vi "Execute.vi"(4 "Position":i32, 6 "Assembly Type":string, 8 "Error In":errorcluster, 9 "Workspace":T1, 10 "Control In":T2={"I-O.lvclass"=refnum, "Gantry"=refnum, "Dispenser"="COM1"}, 11 "Dispense in":refnum<class "Dispense.lvclass">) -> (0 "Error Out":errorcluster, 2 "Control Out":T2={"I-O.lvclass"=refnum, "Gantry"=refnum, "Dispenser"="COM1"}, 3 "Dispense out":refnum<class "Dispense.lvclass">)   [LabVIEW 2021, in "Dispense.lvclass"]
uses:
  Dispense.lvclass
  Controller/Controllers.ctl
  Controller/I-O/I-O.lvclass
  C:/Program Files (x86)/Aerotech/A3200/LabVIEW/2010/Bin/Aerotech.A3200.dll
  Program Files (x86)/Aerotech/A3200/LabVIEW/2010/Bin/Aerotech.A3200.dll
  Workspace/Workspace.ctl
  Dispense.lvclass/Dispense.ctl
  Controller/Controller.lvclass
  Workspace/Fixture.lvclass
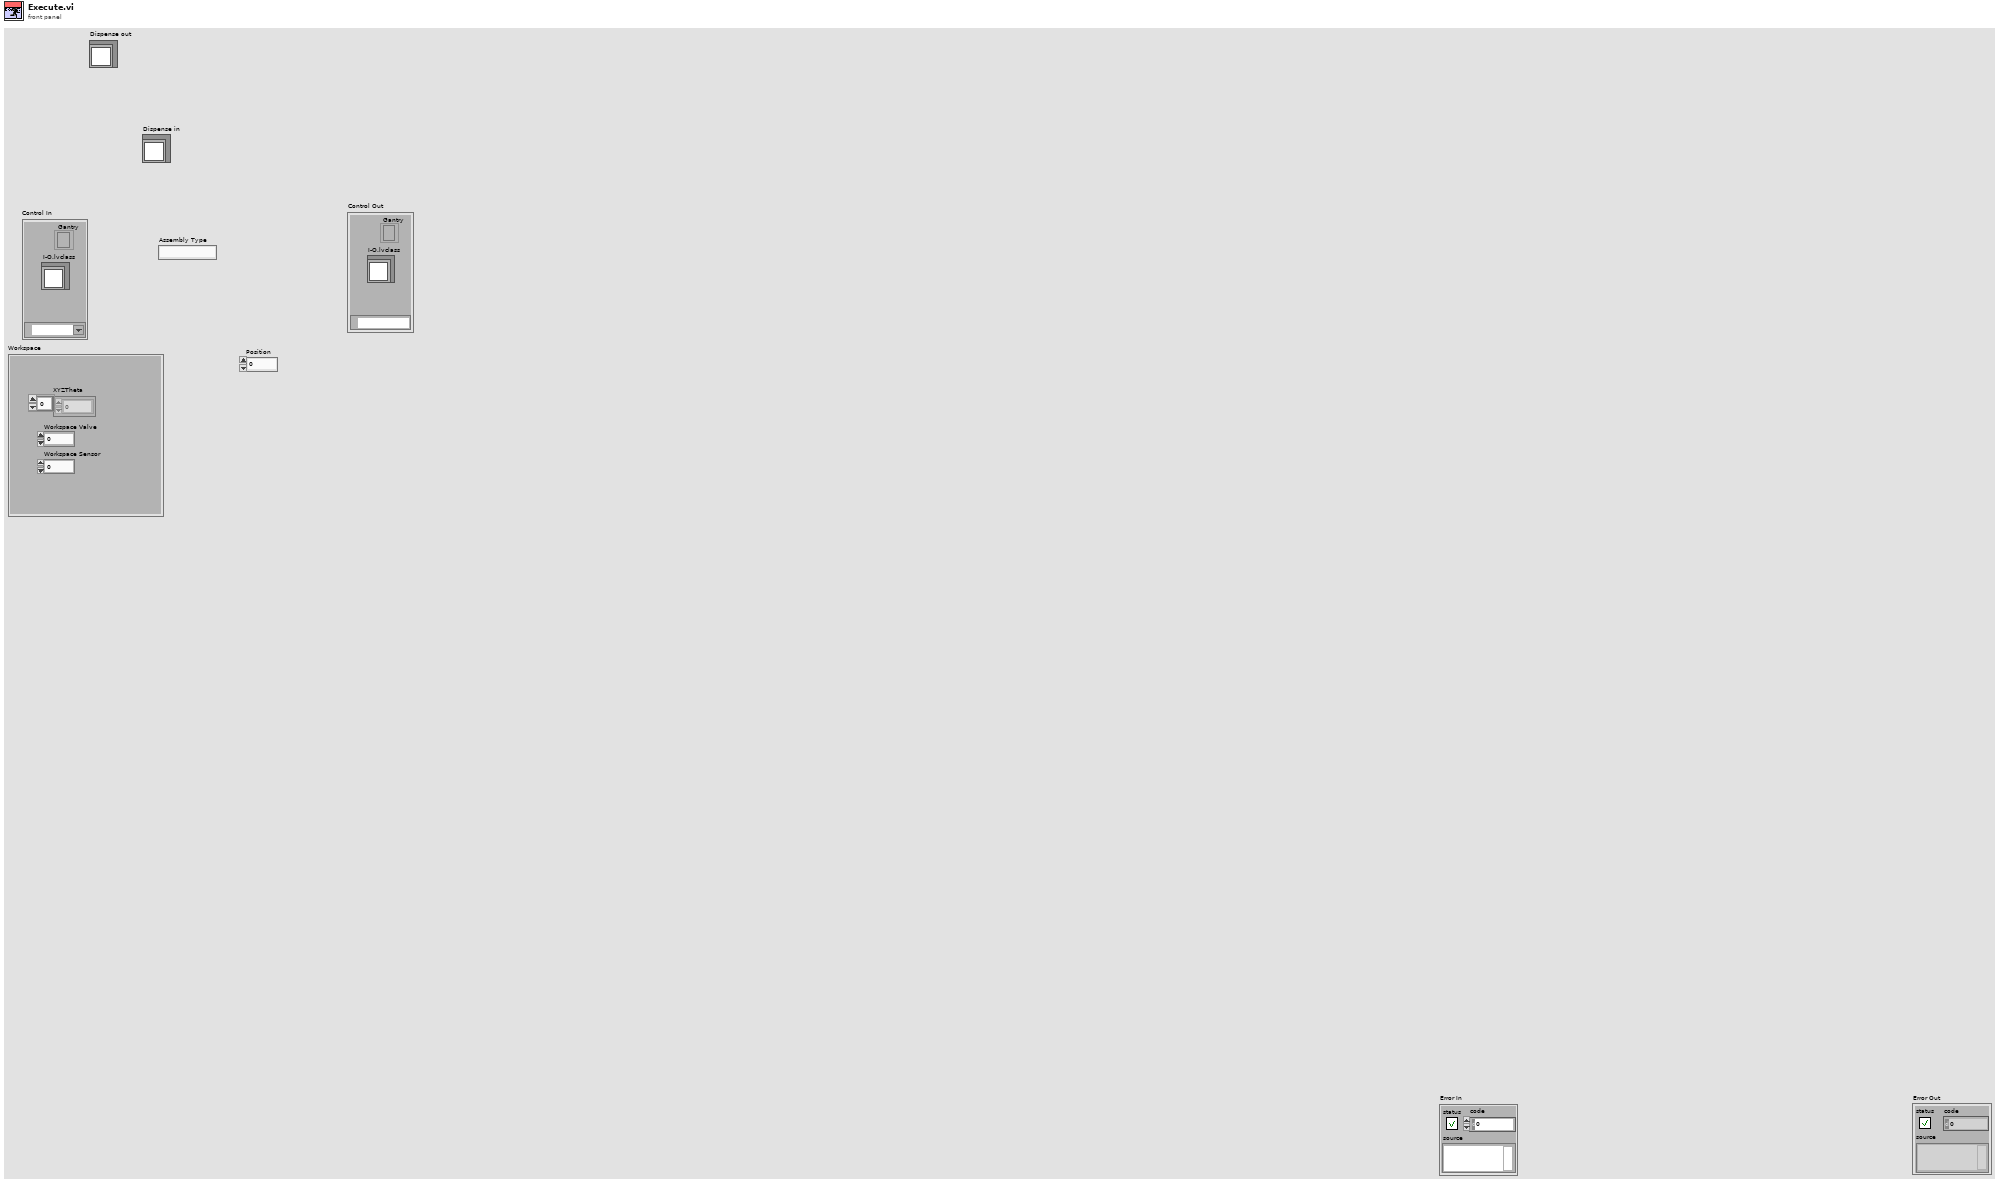
[diagram p1: front panel]
types:
  T1 = typedef "Fixture.lvclass/Workspace.ctl" = cluster{"XYZTheta":dbl[], "Workspace Valve":i32, "Workspace Sensor":i32}
  T2 = typedef "Controller.lvclass/Controllers.ctl" = cluster{"I-O.lvclass":refnum<class "I-O.lvclass">, "Gantry":refnum<k24>, "Dispenser":refnum<visa-resource-name>}
  T3 = cluster{"Time to Go Down":i32, "Time to Dispense":i32}[]
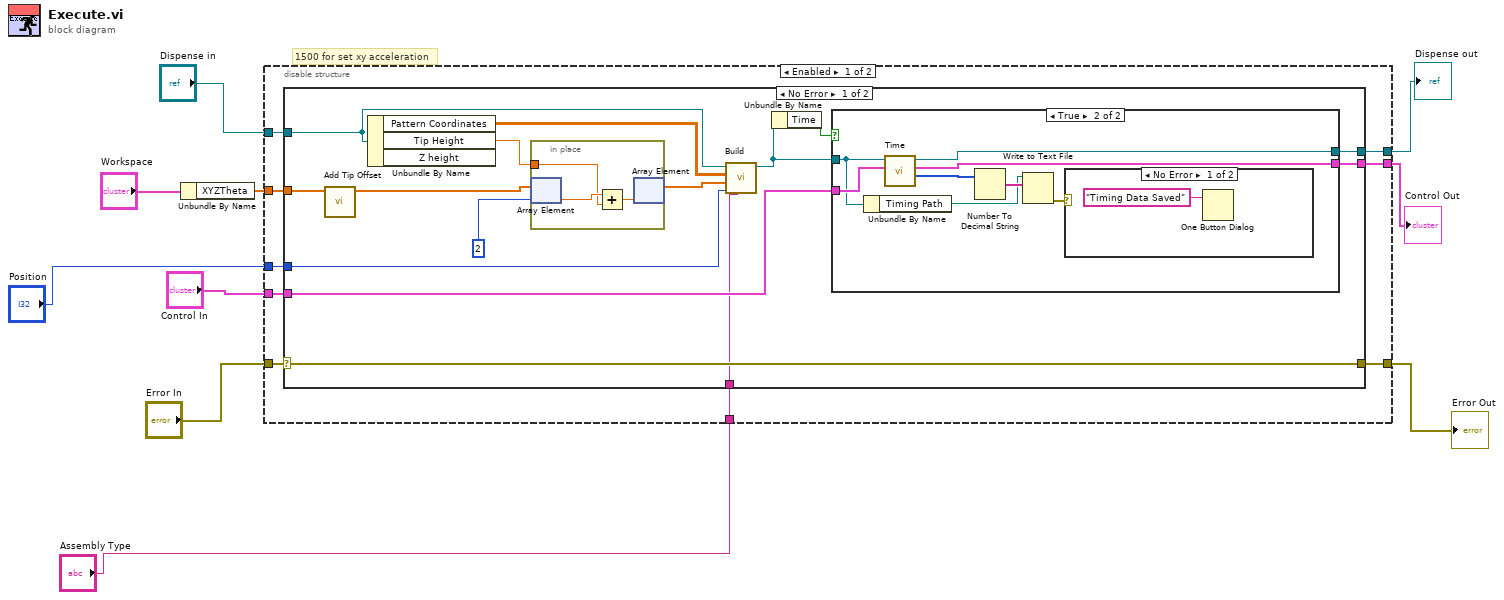
[diagram p0: block diagram]
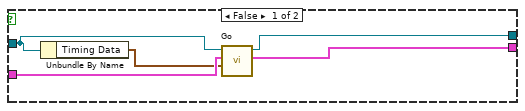
[diagram p2: hidden frame]
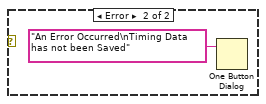
[diagram p3: hidden frame]
diagram:
  # "1500 for set xy acceleration"
  n1 = Unbundle By Name("Workspace") -> ("XYZTheta"=w4:dbl[])
  n2 = disable-structure shown="Enabled" {
    disable-tunnel: "Control In" -> [w19 w56]
    disable-tunnel: [w18 w56] -> w9
    disable-tunnel: "Dispense in" -> [w17 w58]
    disable-tunnel: "Error In" -> [w16 w57]
    disable-tunnel: [w15 w57] -> w6
    disable-tunnel: w4 -> [w14 _]
    disable-tunnel: [w13 w58] -> w3
    disable-tunnel: "Assembly Type" -> [w12 _]
    disable-tunnel: "Position" -> [w11 _]
    frame Enabled {
      n3 = case shown="No Error" w16 {
        selector: w16 -> [w34 w54]
        tunnel: w19 -> [w24 w55]
        tunnel: [w23 w55] -> w18
        tunnel: w17 -> [w27 w53]
        tunnel: [w34 w54] -> w15
        tunnel: w14 -> [w22 _]
        tunnel: [w32 w53] -> w13
        tunnel: w12 -> [w21 _]
        tunnel: w11 -> [w20 _]
        frame No Error {
          n4 = call "Add Tip Offset.vi"("XYZTheta"=w22) -> ("XYZTheta"=w26:dbl[])  [unwired: 10 in]
          n5 = Unbundle By Name(w27) -> ("Pattern Coordinates"=w31:dbl[][], "Tip Height"=w28:dbl)  [unwired: 1 out]
          n6 = in-place {
            in-place-border: w28 -> [w50]
            n7 = in-place-array #1(w26, 2) -> (w52:dbl)
            n8 = Add(x=w52, y=w50) -> (x+y=w51:dbl)
            n9 = in-place-array #1(w51) -> (w29:dbl[])  [unwired: 1 out]
          }
          n10 = call-dynamic "Build.vi"("Assembly Type"=w21, "Position"=w20, "XYZTheta"=w29, "Pattern Coordinates"=w31, "Dispense in"=w27) -> ("Dispense out"=w33:refnum<class "Dispense.lvclass">)  [unwired: 6 in]
          n11 = Unbundle By Name(w33) -> ("Time"=w25:bool)
          n12 = case shown="True" w25 {
            tunnel: w33 -> [w39 w41]
            tunnel: w24 -> [w38 w43]
            tunnel: [w35 w42] -> w23
            tunnel: [w36 w40] -> w32
            frame False {
              n13 = Unbundle By Name(w39) -> ("Timing Data"=w37:T3)
              n14 = call-dynamic "Go.vi"("Timing Data"=w37, "Control In"=w38, "Dispense in"=w39) -> ("Control Out"=w35:T2, "Dispense Out"=w36:refnum<class "Dispense.lvclass">)  [unwired: 7 in]
            }
            frame True {
              n15 = Unbundle By Name(w41) -> ("Timing Path"=w45:path)
              n16 = call-dynamic "Time.vi"("Control In"=w43, "Dispense in"=w41) -> ("Timing Data"=w44:i32[], "Control Out"=w42:T2, "Dispense out"=w40:refnum<class "Dispense.lvclass">)  [unwired: 6 in, 1 out]
              n17 = Number To Decimal String(number=w44) -> (decimal integer string=w46:string[])  [unwired: 1 in]
              n18 = Write to Text File(file (use dialog)=w45, text=w46) -> (error out=w47:errorcluster)  [unwired: 2 in, 2 out]
              n19 = case shown="No Error" w47 {
                frame No Error {
                  n20 = One Button Dialog(message="Timing Data Saved") -> ()  [unwired: 1 in, 1 out]
                }
                frame Error {
                  n21 = One Button Dialog(message="An Error Occurred\nTiming Data has not been Saved") -> ()  [unwired: 1 in, 1 out]
                }
              }
            }
          }
        }
        frame Error {
        }
      }
    }
    frame Disabled {
    }
  }
  "Control Out" <- w9
  "Error Out" <- w6
  "Dispense out" <- w3
